vi "Configure Trigger Event SMU Measure.vi"(0 "VISA resource name":refnum<visa-resource-name>, 5 "Source Measure Unit Channel (0: Channel A)":i32(ring) items=["Channel A", "Channel B"], 7 "Event ID":string, 11 "error in (no error)":errorcluster) -> (4 "VISA resource name out":refnum<visa-resource-name>, 15 "error out":errorcluster)   [LabVIEW 2019, in "Keithley 2600 Series.lvlib"]
doc: "Configures the event that will cause the measure event detector to enter the detected state."
uses:
  Keithley 2600 Series.lvlib
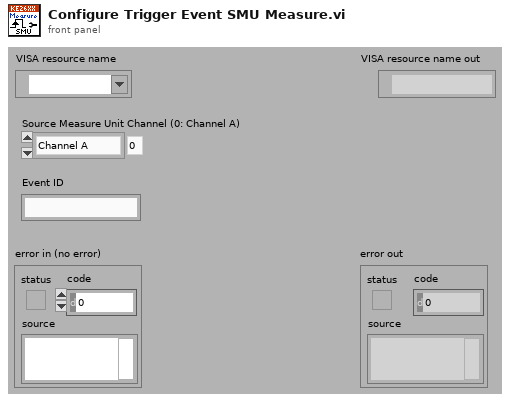
[diagram p1: front panel]
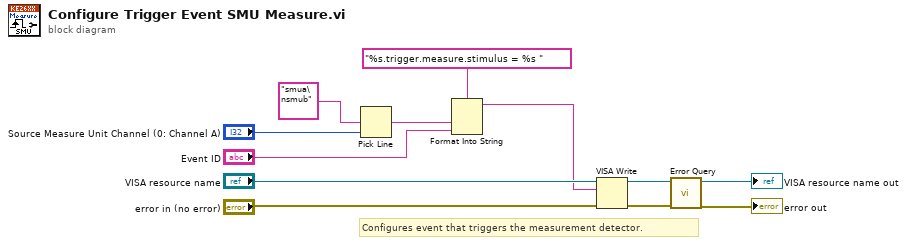
[diagram p0: block diagram]
diagram:
  # "Configures event that triggers the measurement detector."
  n1 = Pick Line(multi-line string="smua\nsmub", line index="Source Measure Unit Channel (0: Channel A)") -> (output string=w3:string)  [unwired: 1 in]
  n2 = Format Into String(format string="%s.trigger.measure.stimulus = %s ", w3, "Event ID") -> (resulting string=w1:string)  [unwired: 2 in, 1 out]
  n3 = VISA Write(VISA resource name="VISA resource name", write buffer=w1, error in (no error)="error in (no error)") -> (VISA resource name out=w9:refnum<visa-resource-name>, error out=w8:errorcluster)  [unwired: 1 out]
  n4 = call "Error Query.vi"("error in (no error)"=w8, "VISA resource name"=w9) -> ("error out"=→"error out":errorcluster, "VISA resource name out"=→"VISA resource name out":refnum<visa-resource-name>)  [unwired: 6 in, 2 out]
